vi "Send Set DER SetPointV Msg.vi"(8 "error in":errorcluster, 10 "DER_SetPointV":T1, 11 "SCADA Sub Abstract in":refnum<class "Device Communication and Control Abstract.lvclass">) -> (0 "error out":errorcluster, 3 "dup SCADA Sub Abstract":refnum<class "Device Communication and Control Abstract.lvclass">)   [LabVIEW 2018, in "Device Communication and Control Abstract Actor.lvlib" / "Device Communication and Control Abstract.lvclass"]
uses:
  Device Communication and Control Abstract.lvclass
  C:/Program Files (x86)/National Instruments/LabVIEW 2018/vi.lib/ActorFramework/Actor/Actor.lvclass
  <vilib>/ORNL/CSEISMIC DDS/CSEISMIC DDS Base/Data Types/DER_SetPointV.ctl
  <vilib>/ORNL/CSEISMIC DDS/CSEISMIC DDS Base/Data Types/Controls/DeviceID.ctl
  <vilib>/ActorFramework/Actor/Actor.lvclass/Actor.ctl
  Device Communication and Control Abstract.lvclass/Device Communication and Control Abstract.ctl
  Device Communication and Control Abstract Messages/Set DER SetPointV Msg/Set DER SetPointV Msg.lvclass/Set DER SetPointV Msg.ctl
  <vilib>/ActorFramework/Message Enqueuer/Message Enqueuer.lvclass/Message Enqueuer.ctl
  <vilib>/ActorFramework/Message Enqueuer/Enqueue.vi
  Device Communication and Control Abstract Messages/Set DER SetPointV Msg/Set DER SetPointV Msg.lvclass
  C:/Program Files (x86)/National Instruments/LabVIEW 2018/vi.lib/ActorFramework/Message/Message.lvclass
  <vilib>/ActorFramework/Message Priority Queue/Priority Enqueue.vi
  <vilib>/ActorFramework/Actor/Actor.lvclass
  <vilib>/ORNL/CSEISMIC DDS/CSEISMIC DDS Base/CSEISMIC DDS.lvclass
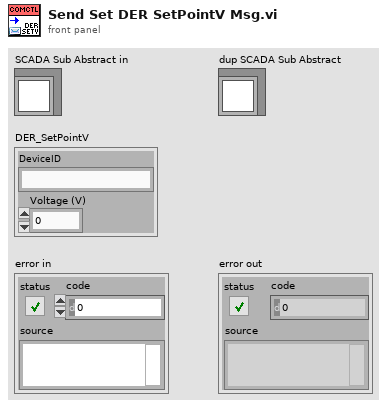
[diagram p1: front panel]
types:
  T1 = typedef "CSEISMIC DDS.lvlib/CSEISMIC DDS.lvclass/DER_SetPointV.ctl" = cluster{"DeviceID":T2, "Voltage (V)":dbl}
  T2 = typedef "CSEISMIC DDS.lvlib/CSEISMIC DDS.lvclass/DeviceID.ctl" = string
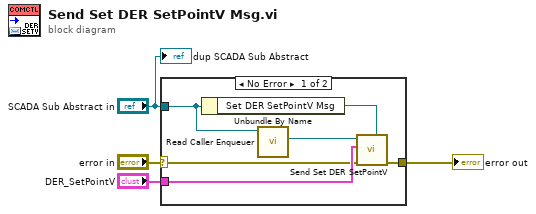
[diagram p0: block diagram]
diagram:
  n1 = case shown="No Error" "error in" {
    selector: "error in" -> [w6 w11]
    tunnel: "SCADA Sub Abstract in" -> [w8 _]
    tunnel: "DER_SetPointV" -> [w7 _]
    tunnel: [w5 w11] -> w1
    frame No Error {
      n2 = Unbundle By Name(w8) -> ("Set DER SetPointV Msg"=w9:refnum<class "Set DER SetPointV Msg.lvclass">)
      n3 = call <vilib>:"Read Caller Enqueuer.vi"("Actor"=w8) -> ("Caller Enqueuer"=w10:refnum<class "Message Enqueuer.lvclass">)  [unwired: 10 in]
      n4 = call "Send Set DER SetPointV.vi"("Message Type"=w9, "error in (no error)"=w6, "DER_SetPointV"=w7, "Message Enqueuer"=w10) -> ("error out"=w5:errorcluster)  [unwired: 6 in, 1 out]
    }
    frame Error {
    }
  }
  "error out" <- w1
  "dup SCADA Sub Abstract" <- "SCADA Sub Abstract in"
